vi "Calibrate XY.vi"(8 "error constant":errorcluster, 11 "Modules":refnum<class "Module.lvclass">[](array[class])) -> (3 "Continue?":bool)   [LabVIEW 2020, in "Module.lvclass"]
uses:
  Module.lvclass
panel:
  out "Y":cluster{i32[], dbl[]}[](graph)
  out "X":cluster{i32[], dbl[]}[](graph)
  in  "Move On":bool
  in  "Again":bool
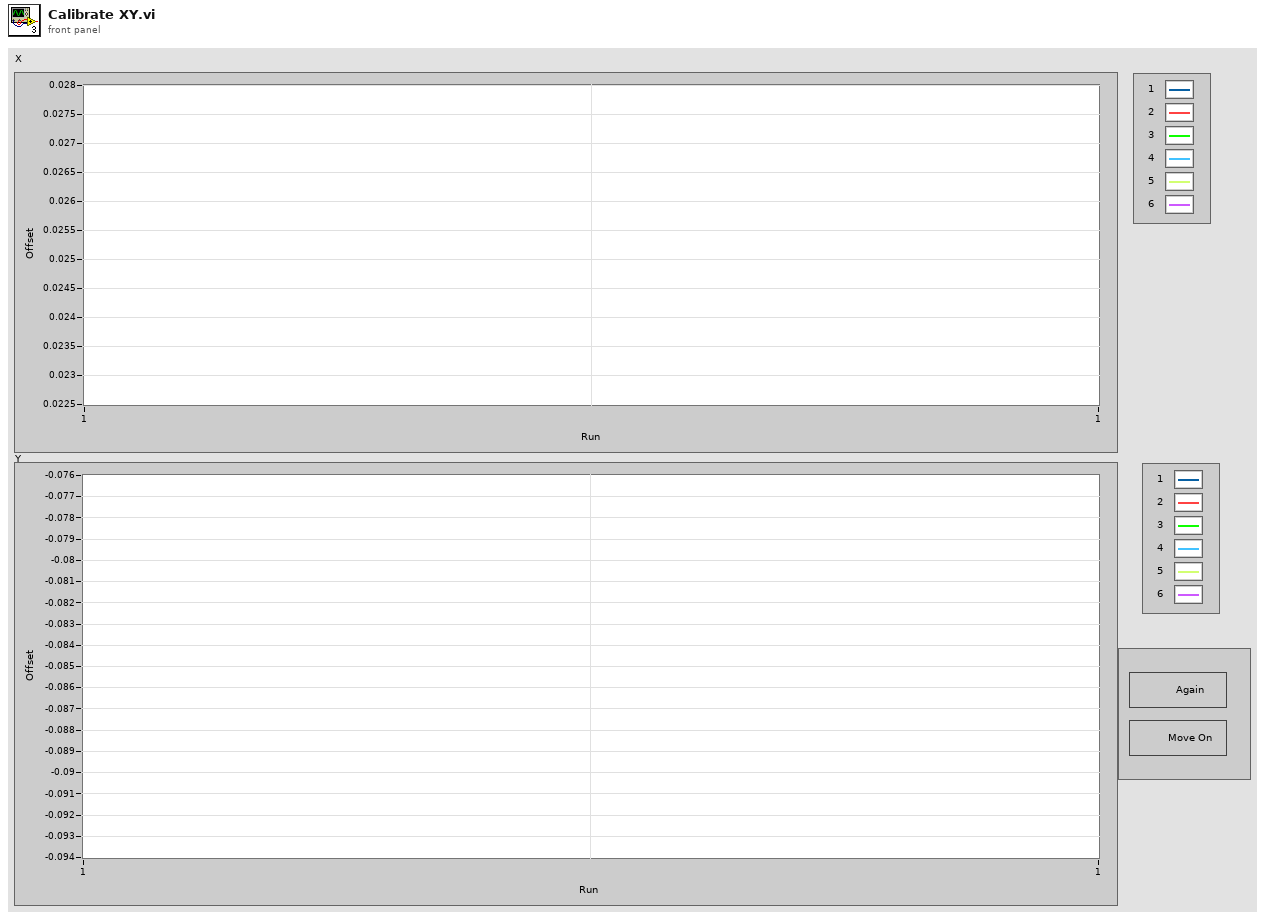
[diagram p1: front panel]
types:
  T1 = enum32{"Invalid", "Standard", "Closed", "Hidden", "Minimized", "Maximized"}
  T2 = typedef "File Paths.ctl" = cluster{"Glue Pattern Folder":path, "Carrier Tray Folder":path, "Pick Up Tool Fixture Folder":path, "Components Folder":path, "Bellows Tool Offset.txt":path, "Pick Up Tool Offset.txt":path, "Dispense Tip Offset.txt":path, "Log Files":path, "Gantry Assembly Map.txt":path, "Syringe and offset map.txt":path}
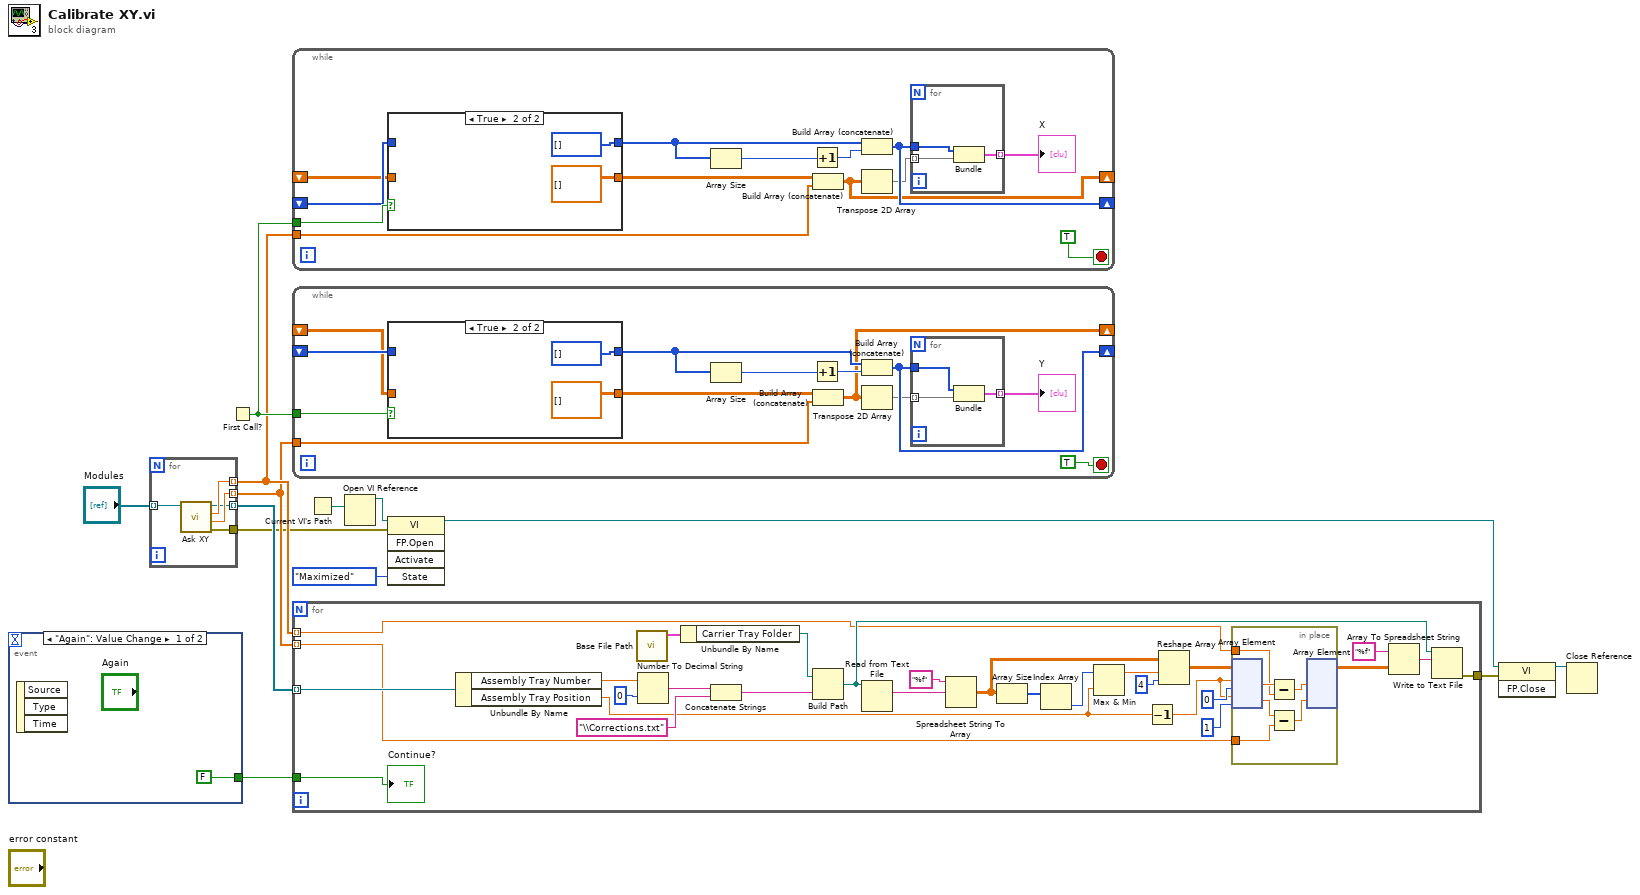
[diagram p0: block diagram]
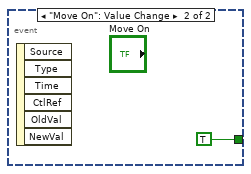
[diagram p4: hidden frame]
diagram:
  n1 = event shown="[0] \"Again\": Value Change" {
    selector: _ -> [_ _]
    dyn-events: _ -> [_ _]
    timeout: _ -> [_ _]
    tunnel: [FALSE TRUE] -> w12
    event "Again": Value Change {
      n2 = event-data() -> ()  [unwired: 1 in, 3 out]
    }
    event "Move On": Value Change {
      n3 = event-data() -> ()  [unwired: 1 in, 6 out]
    }
  }
  n4 = for {
    tunnel: "Modules" -> [w20] mode=indexing
    tunnel: [w19] -> w9 mode=indexing
    tunnel: [w18] -> w8 mode=indexing
    tunnel: [w17] -> w10 mode=indexing
    tunnel: [w16] -> w6
    n5 = call "Ask XY.vi"("Module in"=w20) -> ("error out"=w16:errorcluster, "Y Error Out"=w18:dbl, "X Error Out"=w19:dbl, "Module out"=w17:refnum<class "Module.lvclass">)  [unwired: 7 in]
  }
  n6 = First Call?() -> (First Call?: T/F=w11:bool)
  n7 = while {
    tunnel: w9 -> [w32]
    tunnel: w11 -> [w33]
    shift-right: [w23] -> _
    shift-left: _ -> [w28]
    shift-right: [w24] -> _
    shift-left: _ -> [w31]
    stop <- TRUE stop-if-true
    n8 = case shown="True" w33 {
      tunnel: [w37 i32[] []] -> w25
      tunnel: w31 -> [w37 _]
      tunnel: [w38 dbl[][] []] -> w29
      tunnel: w28 -> [w38 _]
      frame False {
      }
      frame True {
      }
    }
    n9 = Array Size(array=w25) -> (size(s)=w26:i32)
    n10 = Increment(x=w26) -> (x+1=w27:i32)
    n11 = Build Array (concatenate)(w29, w32) -> (w23:dbl[][])
    n12 = Build Array (concatenate)(w25, w27) -> (w24:i32[])
    n13 = Transpose 2D Array(2D array=w23) -> (transposed array=w22:dbl[][])
    n14 = for {
      tunnel: w22 -> [w34] mode=indexing
      tunnel: [w36] -> w21 mode=indexing
      tunnel: w24 -> [w35]
      n15 = Bundle(w35, w34) -> (w36:cluster{i32[], dbl[]})  [unwired: 1 in]
    }
    "X" <- w21
  }
  n16 = while {
    tunnel: w8 -> [w52]
    tunnel: w11 -> [w53]
    shift-right: [w43] -> _
    shift-left: _ -> [w48]
    shift-right: [w44] -> _
    shift-left: _ -> [w51]
    stop <- TRUE stop-if-true
    n17 = case shown="True" w53 {
      tunnel: [w57 i32[] []] -> w45
      tunnel: w51 -> [w57 _]
      tunnel: [w58 dbl[][] []] -> w49
      tunnel: w48 -> [w58 _]
      frame False {
      }
      frame True {
      }
    }
    n18 = Array Size(array=w45) -> (size(s)=w46:i32)
    n19 = Increment(x=w46) -> (x+1=w47:i32)
    n20 = Build Array (concatenate)(w49, w52) -> (w43:dbl[][])
    n21 = Build Array (concatenate)(w45, w47) -> (w44:i32[])
    n22 = Transpose 2D Array(2D array=w43) -> (transposed array=w42:dbl[][])
    n23 = for {
      tunnel: w42 -> [w54] mode=indexing
      tunnel: [w56] -> w41 mode=indexing
      tunnel: w44 -> [w55]
      n24 = Bundle(w55, w54) -> (w56:cluster{i32[], dbl[]})  [unwired: 1 in]
    }
    "Y" <- w41
  }
  n25 = for {
    tunnel: w12 -> [w74]
    tunnel: w10 -> [w73] mode=indexing
    tunnel: w9 -> [w71] mode=indexing
    tunnel: w8 -> [w70] mode=indexing
    tunnel: [w69] -> w2
    n26 = Unbundle By Name(w73) -> ("Assembly Tray Number"=w72:dbl, "Assembly Tray Position"=w63:dbl)
    n27 = call "Base File Path.vi"() -> ("Paths Out"=w80:T2)  [unwired: 11 in]
    n28 = Number To Decimal String(number=w72, width (-)=i16 0) -> (decimal integer string=w83:string)
    n29 = Unbundle By Name(w80) -> ("Carrier Tray Folder"=w81:path)
    n30 = Concatenate Strings(w83, "\\Corrections.txt" ("string")) -> (w85:string)
    n31 = Build Path(base path=w81, name or relative path=w85) -> (appended path=w88:path)
    n32 = Read from Text File(file (use dialog)=w88) -> (text=w86:string)  [unwired: 3 in, 3 out]
    n33 = Spreadsheet String To Array(format string="%f", spreadsheet string=w86) -> (array=w67:dbl[][])  [unwired: 2 in]
    n34 = Array Size(array=w67) -> (size(s)=w66:i32[])
    n35 = Index Array(array=w66) -> (element=w65:i32)  [unwired: 1 in]
    n36 = Max & Min(x=w65, y=w63) -> (max(x,y)=w62:dbl)  [unwired: 1 out]
    n37 = Decrement(x=w63) -> (x-1=w64:dbl)
    n38 = Reshape Array(w67, w62, 4 ("dimension size")) -> (w61:dbl[][])
    n39 = in-place {
      in-place-border: w71 -> [w93]
      in-place-border: w70 -> [w90]
      n40 = in-place-array #1(w61, w64, 0 ("disabled index (col)"), w64, 1 ("disabled index (col)")) -> (w94:dbl, w91:dbl)
      n41 = Subtract(x=w94, y=w93) -> (x-y=w92:dbl)
      n42 = Subtract(x=w91, y=w90) -> (x-y=w89:dbl)
      n43 = in-place-array #1(w92, w89) -> (w77:dbl[][])  [unwired: 4 out]
    }
    n44 = Array To Spreadsheet String(array=w77, 3:"%f" ("format string")) -> (spreadsheet string=w76:string)  [unwired: 1 in]
    n45 = Write to Text File(file (use dialog)=w88, text=w76) -> (error out=w69:errorcluster)  [unwired: 2 in, 2 out]
    "Continue?" <- w74
  }
  n46 = Current VI's Path() -> (path=w7:path)
  n47 = Open VI Reference(vi path=w7) -> (vi reference=w3:refnum<vi>)  [unwired: 5 in, 1 out]
  n48 = invoke class="VI" method="FP.Open"(reference=w3, error in=w6, "State"=T1."Maximized") -> (reference out=w4:refnum<vi>)  [unwired: 2 in, 4 out]
  n49 = invoke class="VI" method="FP.Close"(reference=w4, error in=w2) -> (reference out=w1:refnum<vi>)  [unwired: 1 in, 2 out]
  n50 = Close Reference(reference=w1) -> ()  [unwired: 1 in, 1 out]
